vi "Actor Core.vi"(8 "error in":errorcluster, 11 "Nested in":refnum<class "Chart Actor.lvclass">) -> (0 "error out":errorcluster, 3 "Actor out":refnum<class "Actor.lvclass">)   [LabVIEW 2018, in "Chart Actor.lvlib" / "Chart Actor.lvclass"]
doc: "(<B>Filename</B>: Actor Framework.lvlib:Actor.lvclass:Actor Core.vi)\n\nReceives messages to the actor, reacts to them, and initiates any error handling that may shut the actor down.\n\nDescendant classes may override this VI to append parallel tasks for the actor to complete while it handles messages. Overrides use the Call Parent Method node."
uses:
  Chart Actor.lvclass
  D:/Program Files (x86)/National Instruments/LabVIEW 2018/vi.lib/MGI/Panel Manager/Panel Actor/Panel Actor/Panel Actor.lvclass
  <vilib>/ActorFramework/Actor/Actor.lvclass
  Chart Actor.lvclass/Chart Actor.ctl
  Chart Actor Messages/1 UpdateChartData Msg/1 UpdateChartData Msg.lvclass
  D:/Program Files (x86)/National Instruments/LabVIEW 2018/vi.lib/ActorFramework/Message/Message.lvclass
  <vilib>/ActorFramework/Message Enqueuer/Message Enqueuer.lvclass/Message Enqueuer.ctl
  <vilib>/ActorFramework/Message Enqueuer/Enqueue.vi
  <vilib>/ActorFramework/Stop Msg/Stop Msg.lvclass
  <vilib>/ActorFramework/Message Priority Queue/Priority Enqueue.vi
  <vilib>/MGI/Panel Manager/Panel Actor/Panel Actor/Panel Actor.lvclass
panel:
  out "波形图表":dbl(graph)
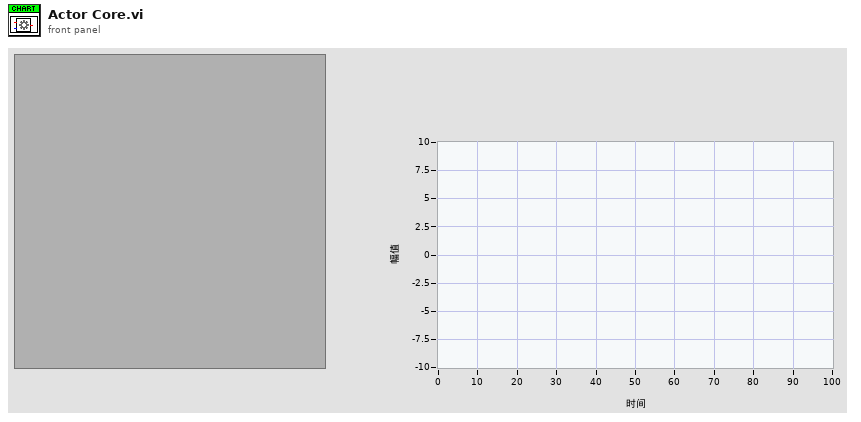
[diagram p1: front panel]
types:
  T1 = cluster{"事件注册引用句柄":refnum<event-registration>, "Pnl Actor":refnum<event-registration>}
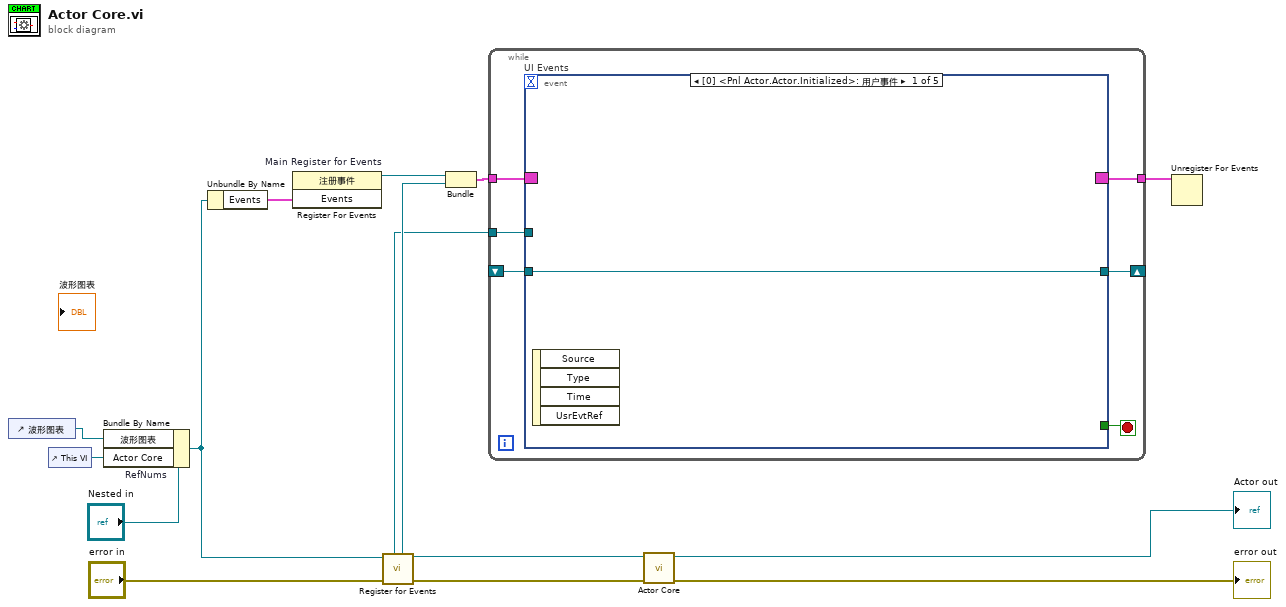
[diagram p0: block diagram]
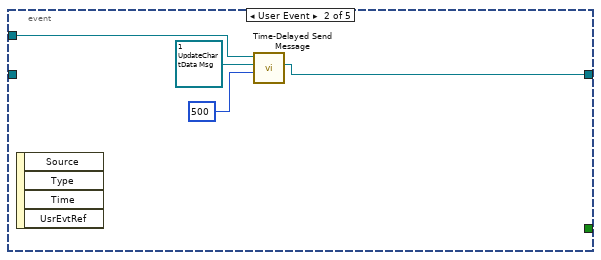
[diagram p2: hidden frame]
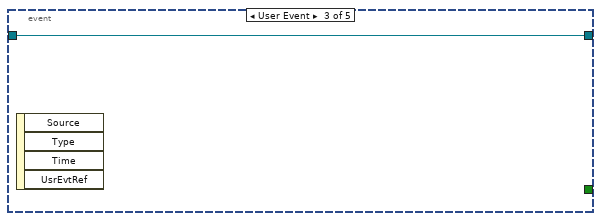
[diagram p3: hidden frame]
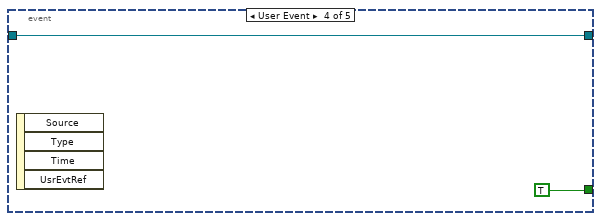
[diagram p4: hidden frame]
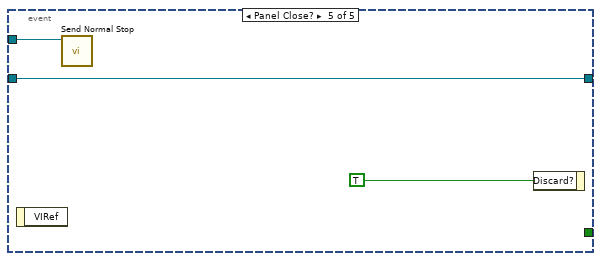
[diagram p5: hidden frame]
diagram:
  n1 = control-ref of="波形图表"() -> (w2:refnum<vi>)
  n2 = control-ref of="This VI"() -> (w10:refnum<vi>)
  n3 = Bundle By Name "RefNums"(cluster="Nested in", "波形图表"=w2, "Actor Core"=w10) -> (w9:refnum<class "Chart Actor.lvclass">)
  n4 = Unbundle By Name(w9) -> ("Events"=w13:cluster{"Stop":refnum<user-event>})
  n5 = register-events "Main Register for Events"(w13) -> (reference out=w5:refnum<event-registration>)  [unwired: 2 in, 1 out]
  n6 = call <vilib>:"Register for Events.vi"("Error In"="error in", "Panel Actor in"=w9) -> ("Error Out"=w6:errorcluster, "Panel Actor out"=w8:refnum<class "Chart Actor.lvclass">, "Pnl Actor"=w3:refnum<event-registration>, "Self Enqueuer"=w1:refnum<class "Message Enqueuer.lvclass">)  [unwired: 6 in]
  n7 = Bundle("事件注册引用句柄"=w5, "Pnl Actor"=w3) -> (w4:T1)  [unwired: 1 in]
  n8 = while {
    tunnel: w4 -> [w21]
    tunnel: [w19] -> w12
    tunnel: w1 -> [w18]
    shift-right: [w17] -> _
    shift-left: _ -> [w16]
    stop <- w20 stop-if-true
    n9 = event "UI Events" shown="[0] <Pnl Actor.Actor.Initialized>: 用户事件" {
      selector: w21 -> [_ _ _ _ _]
      dyn-events: [_ _ _ _ _] -> w19
      timeout: _ -> [_ _ _ _ _]
      tunnel: [_ _ _ TRUE _] -> w20
      tunnel: w18 -> [_ w24 _ _ w31]
      tunnel: [w22 w23 w27 w28 w30] -> w17
      tunnel: w16 -> [w22 _ w27 w28 w30]
      event User Event {
        n10 = event-data() -> ()  [unwired: 1 in, 4 out]
      }
      event User Event {
        n11 = event-data() -> ()  [unwired: 1 in, 4 out]
        n12 = call <vilib>:"Time-Delayed Send Message.vi"("Milliseconds To Wait"=500, "Message"=refnum<class "1 UpdateChartData Msg.lvclass"> refnum ("Chart Actor.lvlib:1 UpdateChartData Msg.lvclass"), "Message Enqueuer"=w24) -> ("Delivery Notifier"=w23:refnum<notifier>)  [unwired: 7 in, 1 out]
      }
      event User Event {
        n13 = event-data() -> ()  [unwired: 1 in, 4 out]
      }
      event User Event {
        n14 = event-data() -> ()  [unwired: 1 in, 4 out]
      }
      event Panel Close? {
        n15 = event-data() -> ()  [unwired: 1 in, 1 out]
        n16 = call <vilib>:"Send Normal Stop.vi"("Message Enqueuer"=w31) -> ()  [unwired: 10 in, 1 out]
        n17 = event-data("Discard?"=TRUE) -> ()  [unwired: 1 in, 1 out]
      }
    }
  }
  n18 = call-parent "Actor Core.vi"("error in"=w6, "Panel Actor in"=w8) -> ("error out"=→"error out":errorcluster, "Actor out"=→"Actor out":refnum<class "Actor.lvclass">)  [unwired: 8 in]
  n19 = Unregister For Events(event registration refnum=w12) -> ()  [unwired: 1 in, 1 out]
